vi "UpdateEngine.vi"(8 "error in (no error)":errorcluster, 11 "Pump_1AI_1DO_2DI in":refnum<class "Engine_1DO_2DI.lvclass">) -> (0 "error out":errorcluster, 3 "Pump_1AI_1DO_2DI out":refnum<class "Engine_1DO_2DI.lvclass">)   [LabVIEW 2019, in "Engine_1DO_2DI.lvclass"]
uses:
  Engine_1DO_2DI.lvclass
  D:/GIT H4000/H4000/src/Device_class/Device.lvclass
  D:/GIT H4000/H4000/src/Proccess_class/Proccess.lvclass
  Device_class/Device.lvclass/Device.ctl
  Engine_1DO_2DI.lvclass/Engine_1DO_2DI.ctl
  TypeDef/State Engine.ctl
  DA_class/DA.lvclass/DA.ctl
  Proccess_class/Proccess.lvclass/Proccess.ctl
  subvis/bool_change.vi
  DA_class/private/write_to_db.vi
  Proccess_class/GetNames.vi
  Proccess_class/GetLogger.vi
  private/SendToDb.vi/c0b53383-3d34-4a55-8dce-306f7f934b6c.vi
  DA_class/DA.lvclass
  Logger_class/WriteEvent.vi
  FPGA_API_class/FPGA API.lvclass
  Device_class/Device.lvclass
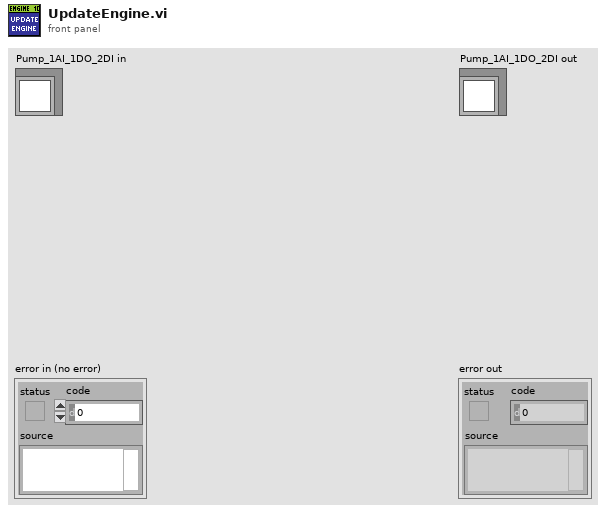
[diagram p1: front panel]
types:
  T1 = typedef "State Engine.ctl" = enum16{"Unknown", "Off", "TupningOn", "On", "TurningOff"}
  T2 = typedef "DI index.ctl" = u8
  T3 = typedef "DO index.ctl" = u8
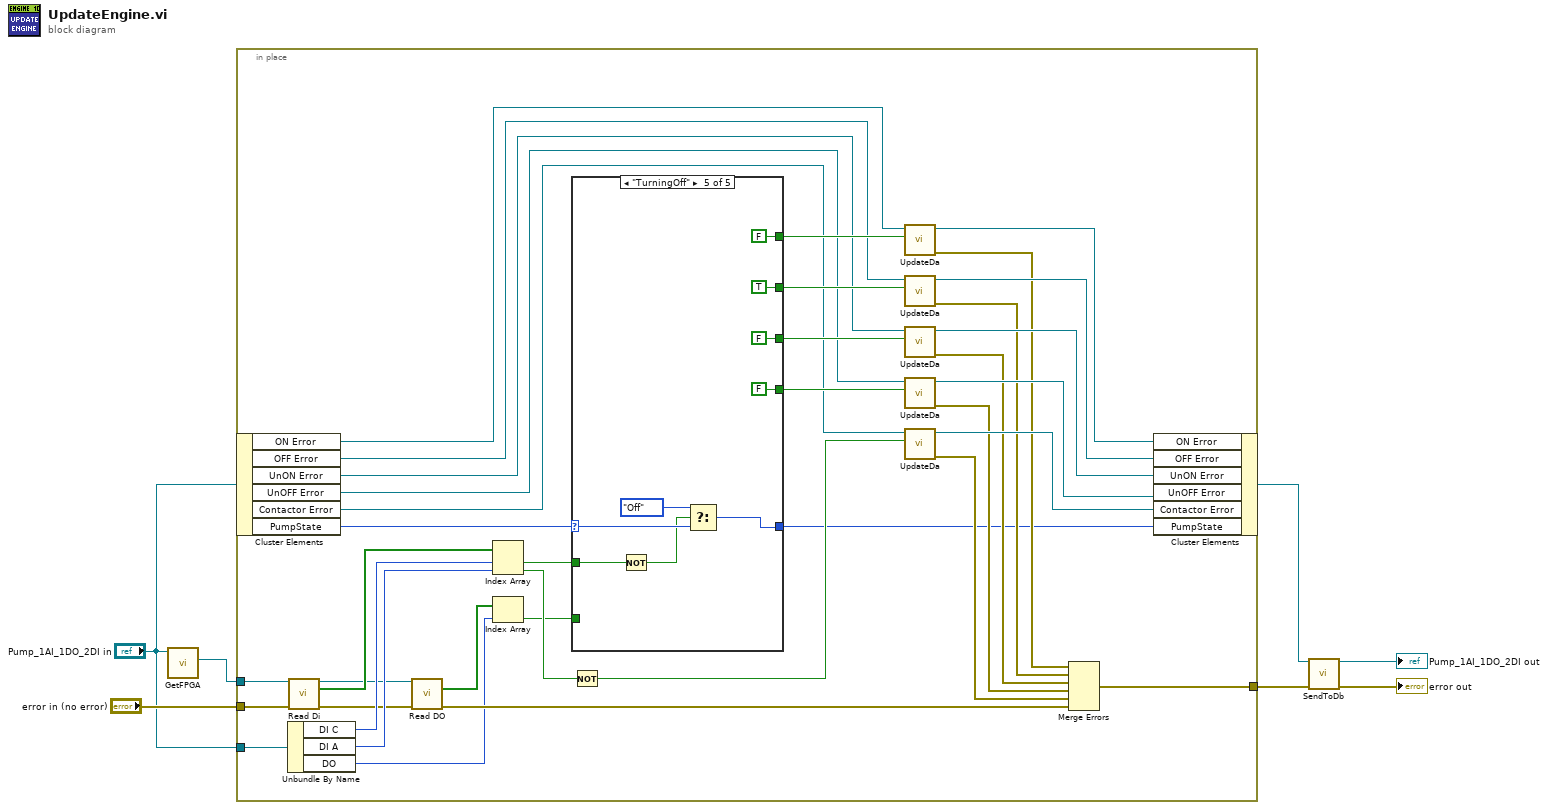
[diagram p0: block diagram]
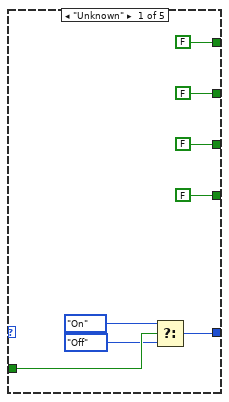
[diagram p2: hidden frame]
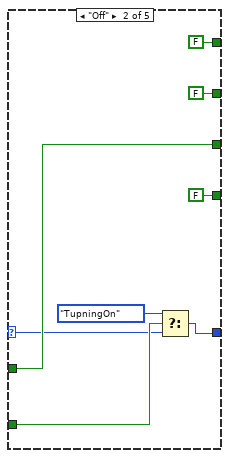
[diagram p3: hidden frame]
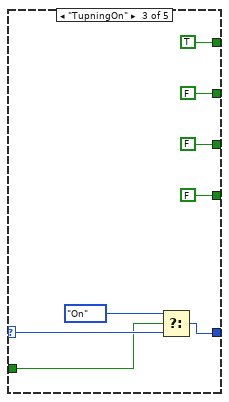
[diagram p4: hidden frame]
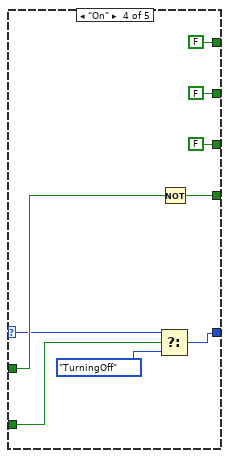
[diagram p5: hidden frame]
diagram:
  n1 = call "GetFPGA.vi"("Device in"="Pump_1AI_1DO_2DI in") -> ("FPGA API.lvclass"=w5:refnum<class "FPGA API.lvclass">)  [unwired: 10 in]
  n2 = in-place {
    in-place-border: "error in (no error)" -> [w39]
    in-place-border: [w44] -> w2
    in-place-border: "Pump_1AI_1DO_2DI in" -> [w43]
    in-place-border: w5 -> [w16]
    n3 = in-place-cluster #1("Pump_1AI_1DO_2DI in") -> ("ON Error"=w26:refnum<class "DA.lvclass">, "OFF Error"=w25:refnum<class "DA.lvclass">, "UnON Error"=w24:refnum<class "DA.lvclass">, "UnOFF Error"=w23:refnum<class "DA.lvclass">, "Contactor Error"=w22:refnum<class "DA.lvclass">, "PumpState"=w9:T1)
    n4 = Unbundle By Name(w43) -> ("DI C"=w41:T2, "DI A"=w40:T2, "DO"=w11:T3)
    n5 = call-dynamic "Read Di.vi"("FPGA API in"=w16, "error in (no error)"=w39) -> ("FPGA API out"=w14:refnum<class "FPGA API.lvclass">, "DIs"=w42:bool[], "error out"=w15:errorcluster)  [unwired: 11 in]
    n6 = call-dynamic "Read DO.vi"("FPGA API in"=w14, "error in (no error)"=w15) -> ("Ds"=w13:bool[], "error out"=w12:errorcluster)  [unwired: 11 in, 1 out]
    n7 = Index Array(array=w42, index #1=w41, index #2=w40) -> (element #1=w38:bool, element #2=w37:bool)
    n8 = Index Array(array=w13, index=w11) -> (element=w10:bool)
    n9 = case shown="\"TurningOff\"" w9 {
      selector: w9 -> [_ w55 w68 w72 w86]
      tunnel: [w49 w53 w66 w70 w84] -> w8
      tunnel: w38 -> [w51 w60 w65 w77 w82]
      tunnel: [FALSE w60 FALSE FALSE FALSE] -> w35
      tunnel: [FALSE ("RAW") FALSE ("RAW") TRUE ("RAW") FALSE ("RAW") FALSE ("RAW")] -> w34
      tunnel: [FALSE ("RAW") FALSE ("RAW") FALSE ("RAW") FALSE ("RAW") TRUE ("RAW")] -> w33
      tunnel: [FALSE ("RAW") FALSE ("RAW") FALSE ("RAW") w76 FALSE ("RAW")] -> w32
      tunnel: w10 -> [_ w56 _ w71 _]
      frame "Unknown" {
        n10 = Select(t=State_Engine."On" ("PumpState"), s=w51, f=State_Engine."Off" ("PumpState")) -> (s? t:f=w49:T1)
      }
      frame "Off" {
        n11 = Select(t=State_Engine."TupningOn", s=w56, f=w55) -> (s? t:f=w53:T1)
      }
      frame "TupningOn" {
        n12 = Select(t=State_Engine."On", s=w65, f=w68) -> (s? t:f=w66:T1)
      }
      frame "On" {
        n13 = Select(t=w72, s=w71, f=State_Engine."TurningOff") -> (s? t:f=w70:T1)
        n14 = Not(x=w77) -> (.not. x?=w76:bool)
      }
      frame "TurningOff" {
        n15 = Not(x=w82) -> (.not. x?=w83:bool)
        n16 = Select(t=State_Engine."Off", s=w83, f=w86) -> (s? t:f=w84:T1)
      }
    }
    n17 = Not(x=w37) -> (.not. x?=w36:bool)
    n18 = call "UpdateDa.vi"("RAW"=w34, "Sig_DA in"=w26) -> ("error out"=w17:errorcluster, "Sig_DA out"=w27:refnum<class "DA.lvclass">)  [unwired: 7 in, 1 out]
    n19 = call "UpdateDa.vi"("RAW"=w33, "Sig_DA in"=w25) -> ("error out"=w18:errorcluster, "Sig_DA out"=w28:refnum<class "DA.lvclass">)  [unwired: 7 in, 1 out]
    n20 = call "UpdateDa.vi"("RAW"=w35, "Sig_DA in"=w24) -> ("error out"=w19:errorcluster, "Sig_DA out"=w29:refnum<class "DA.lvclass">)  [unwired: 7 in, 1 out]
    n21 = call "UpdateDa.vi"("RAW"=w32, "Sig_DA in"=w23) -> ("error out"=w20:errorcluster, "Sig_DA out"=w30:refnum<class "DA.lvclass">)  [unwired: 7 in, 1 out]
    n22 = call "UpdateDa.vi"("RAW"=w36, "Sig_DA in"=w22) -> ("error out"=w21:errorcluster, "Sig_DA out"=w31:refnum<class "DA.lvclass">)  [unwired: 7 in, 1 out]
    n23 = Merge Errors(w17, w18, w19, w20, w21, w12) -> (w44:errorcluster)
    n24 = in-place-cluster #1("ON Error"=w27, "OFF Error"=w28, "UnON Error"=w29, "UnOFF Error"=w30, "Contactor Error"=w31, "PumpState"=w8) -> (w4:refnum<class "Engine_1DO_2DI.lvclass">)
  }
  n25 = call "SendToDb.vi"("reference in"=w4, "error in (no error)"=w2) -> ("reference out"=→"Pump_1AI_1DO_2DI out":refnum<class "Engine_1DO_2DI.lvclass">, "error out"=→"error out":errorcluster)  [unwired: 12 in]
